vi "BotSpeak_RunScript.vi"(2 "Subroutine (runs prgm if unwired)":string, 3 "Bot Settings":T1) -> (0 "response":string="169.254.32.85", 1 "Bot Settings":T1)   [LabVIEW 2012]
doc: "Runs scripted code that has been loaded to the hardware with a Load VI."
uses:
  <userlib>/BotSpeak/VIs/Direct/BotSpeak_Control.ctl
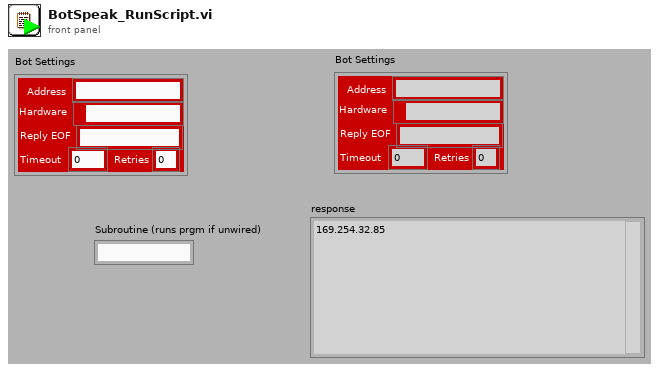
[diagram p1: front panel]
types:
  T1 = typedef "BotSpeak_Control.ctl" = cluster{"Address":string, "Reply EOF":string, "Hardware":path, "Retries":i8, "Timeout":i32}
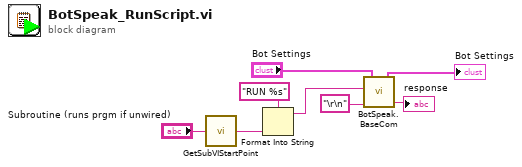
[diagram p0: block diagram]
diagram:
  n1 = call <userlib>:"GetSubVIStartPoint.vi"("Subroutine (runs prgm if unwired)"="Subroutine (runs prgm if unwired)") -> ("String"=w2:string)
  n2 = Format Into String(format string="RUN %s" ("command"), w2) -> (resulting string=w1:string)  [unwired: 2 in, 1 out]
  n3 = call <userlib>:"BotSpeak.BaseCom.vi"("Termination"="\r\n", "command"=w1, "Bot Settings in"="Bot Settings") -> ("response"=→"response":string, "Bot Settings out"=→"Bot Settings":T1)  [unwired: 2 in]
